vi "oa_Check Empty Reset.vi"(10 "empty?":bool, 11 "reset?":bool=TRUE) -> (3 "reset? out":bool)   [LabVIEW 2017, in "SoundVib_Resampling.lvlib"]
uses:
  <vilib>/addons/Sound and Vibration/Order Analysis/Resample Order Tracking/SoundVib_Resampling.lvlib
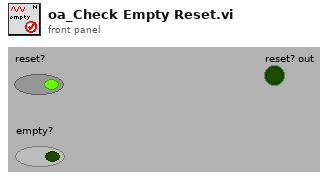
[diagram p1: front panel]
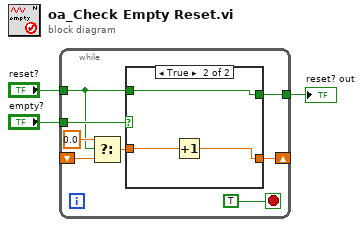
[diagram p0: block diagram]
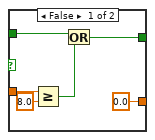
[diagram p2: hidden frame]
diagram:
  n1 = while {
    tunnel: "empty?" -> [w10]
    shift-right: [w6] -> _
    shift-left: _ -> [w8]
    tunnel: "reset?" -> [w5]
    tunnel: [w4] -> w1
    stop <- TRUE stop-if-true
    n2 = Select(t=0.0, s=w5, f=w8) -> (s? t:f=w7:dbl)
    n3 = case shown="True" w10 {
      tunnel: w7 -> [w16 w20]
      tunnel: [0.0 w19] -> w6
      tunnel: w5 -> [w13 w18]
      tunnel: [w12 w18] -> w4
      frame False {
        n4 = Greater Or Equal?(x=w16, y=8.0) -> (x >= y?=w14:bool)
        n5 = Or(x=w13, y=w14) -> (x .or. y?=w12:bool)
      }
      frame True {
        n6 = Increment(x=w20) -> (x+1=w19:dbl)
      }
    }
  }
  "reset? out" <- w1
